vi "PH_gentec_M-Link.set Waveform Averages.vi"(0 "i ref in":refnum<vi>, 2 "VISA resource in":refnum<visa-resource-name>, 5 "error in":errorcluster) -> (11 "Timeout":bool, 13 "Data read":string[](array[string]), 14 "i ref out":refnum<vi>, 16 "VISA resource out":refnum<visa-resource-name>, 17 "Error":bool, 18 "Failure":bool, 19 "error out":errorcluster)   [LabVIEW 2014, in "PH_gentec_M-Link.lvlib"]
doc: "This VI writes wanted Settings to the Device and checks the result."
uses:
  PH_gentec_M-Link.lvlib
  instr.lib/Gentec-M-Link/gentec-M-Link - Driver.lvlib
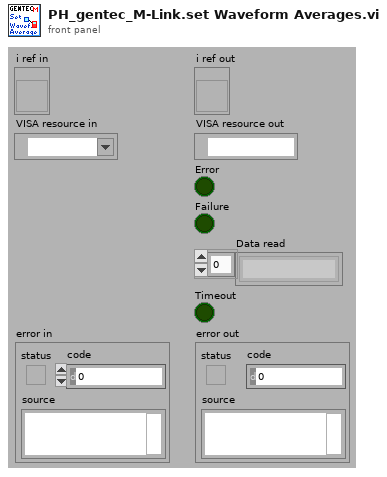
[diagram p1: front panel]
types:
  T1 = typedef "PH_gentec_M-Link.lvlib/PH_gentec_M-Link.i attribute.ctl" = cluster{"GUI References":cluster{"Wanted Head Settings":refnum<vi>, "Current Head Settings":refnum<vi>, "Set Auto Range":refnum<vi>, "Trigger Polarity":refnum<vi>, "Trigger Source":refnum<vi>, "Waveform Averages":refnum<vi>, "Continuous":refnum<vi>, "get one Value":refnum<vi>}, "Wanted Head Settings":T2, "Current Head Settings":T2}
  T2 = typedef "PH_gentec_M-Link.lvlib/PH_gentec_M-Link.Head Settings.ctl" = cluster{"Measurement Mode":T3, "Enable Anticipation":bool, "Set Auto Range":bool, "Block Signal":bool, "Set Head Attenuator":bool, "Enable SSE":bool, "Trigger Polarity":T4, "Trigger Source":T5, "Waveform Averages":T6, "Set Zero":i32, "Current":i32, "Start Data Flow":bool}
  T3 = typedef "gentec-M-Link - Driver.lvlib/gentec-M-Link.Measurement Mode.ctl" = u16
  T4 = typedef "gentec-M-Link - Driver.lvlib/gentec-M-Link.Trigger Polarity.ctl" = u16
  T5 = typedef "gentec-M-Link - Driver.lvlib/gentec-M-Link.Trigger Source.ctl" = u16
  T6 = typedef "gentec-M-Link - Driver.lvlib/gentec-M-Link.Waveform Averages.ctl" = u16
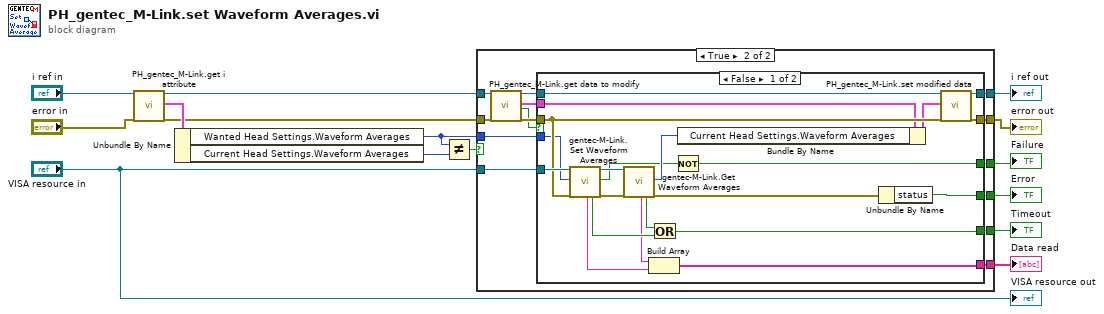
[diagram p0: block diagram]
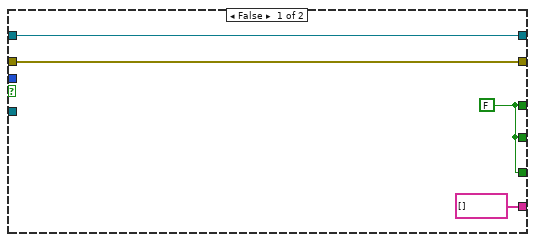
[diagram p2: hidden frame]
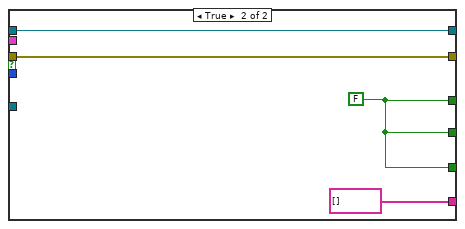
[diagram p3: hidden frame]
diagram:
  n1 = call "PH_gentec_M-Link.get i attribute.vi"("i ref in"="i ref in", "error in (no error)"="error in") -> ("i ref out"=w8:refnum<vi>, "i attribute"=w11:T1, "error out"=w10:errorcluster)  [unwired: 15 in]
  n2 = Unbundle By Name(w11) -> ("Wanted Head Settings.Waveform Averages"=w13:T6, "Current Head Settings.Waveform Averages"=w12:T6)
  n3 = Not Equal?(x=w13, y=w12) -> (x != y?=w1:bool)
  n4 = case shown="True" w1 {
    tunnel: [w16 w33] -> w15
    tunnel: [w17 w32] -> w14
    tunnel: w13 -> [_ w31]
    tunnel: w10 -> [w16 w26]
    tunnel: w8 -> [w17 w25]
    tunnel: "VISA resource in" -> [_ w24]
    tunnel: [w19 w23] -> w5
    tunnel: [w19 w22] -> w4
    tunnel: [w19 w21] -> w3
    tunnel: [string[] [] w20] -> w2
    frame False {
      w19 = FALSE
    }
    frame True {
      n5 = call "PH_gentec_M-Link.get data to modify.vi"("i ref in"=w25, "error in (no error)"=w26) -> ("i ref out"=w29:refnum<vi>, "i attribute"=w28:T1, "timed out"=w27:bool, "error out"=w30:errorcluster)  [unwired: 14 in]
      n6 = case shown="False" w27 {
        tunnel: w24 -> [w53 _]
        tunnel: [w49 w58] -> w32
        tunnel: [w48 w57] -> w33
        tunnel: w30 -> [w52 w57]
        tunnel: w29 -> [w54 w58]
        tunnel: w28 -> [w51 _]
        tunnel: w31 -> [w50 _]
        tunnel: [w46 w56] -> w23
        tunnel: [w34 w56] -> w22
        tunnel: [w45 w56] -> w21
        tunnel: [w44 string[] []] -> w20
        frame False {
          n7 = call "gentec-M-Link.Set Waveform Averages.vi"("VISA resource In"=w53, "Waveform Averages"=w50, "error in (no error)"=w52) -> ("Data Read"=w36:string, "Read Timeout"=w39:bool, "VISA resource Out"=w40:refnum<visa-resource-name>, "Success"=w37:bool, "error out"=w41:errorcluster)  [unwired: 12 in]
          n8 = call "gentec-M-Link.Get Waveform Averages.vi"("VISA resource In"=w40, "error in (no error)"=w41) -> ("Data Read"=w35:string, "Read Timeout"=w38:bool, "Waveform Averages"=w42:T6, "error out"=w43:errorcluster)  [unwired: 13 in, 1 out]
          n9 = Build Array(w35, w36) -> (w44:string[])
          n10 = Or(x=w38, y=w39) -> (x .or. y?=w45:bool)
          n11 = Not(x=w37) -> (.not. x?=w34:bool)
          n12 = Bundle By Name(cluster=w51, "Current Head Settings.Waveform Averages"=w42) -> (w47:T1)
          n13 = Unbundle By Name(w43) -> ("status"=w46:bool)
          n14 = call "PH_gentec_M-Link.set modified data.vi"("i ref in"=w54, "i attribute"=w47, "error in (no error)"=w52) -> ("i ref out"=w49:refnum<vi>, "error out"=w48:errorcluster)  [unwired: 15 in]
        }
        frame True {
          w56 = FALSE
        }
      }
    }
  }
  "error out" <- w15
  "i ref out" <- w14
  "Error" <- w5
  "Failure" <- w4
  "Timeout" <- w3
  "Data read" <- w2
  "VISA resource out" <- "VISA resource in"
